vi "GetAvailableDeviceFamilyNames.vi"(8 "Error in":errorcluster) -> (0 "Error out":errorcluster, 2 "Count":i32, 3 "AvailableDeviceFamilies":string[](array[string]))   [LabVIEW 2016]
doc: "Determines a list of all available device families (device drivers).\n\nAvailableDevices: Array of available device family names\nCount: Number of available device families"
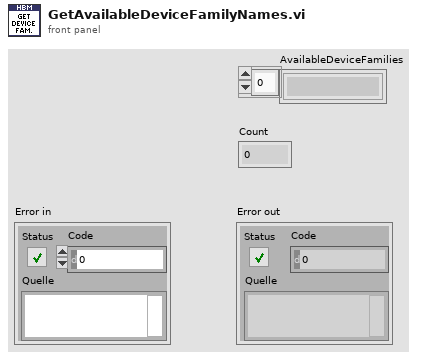
[diagram p1: front panel]
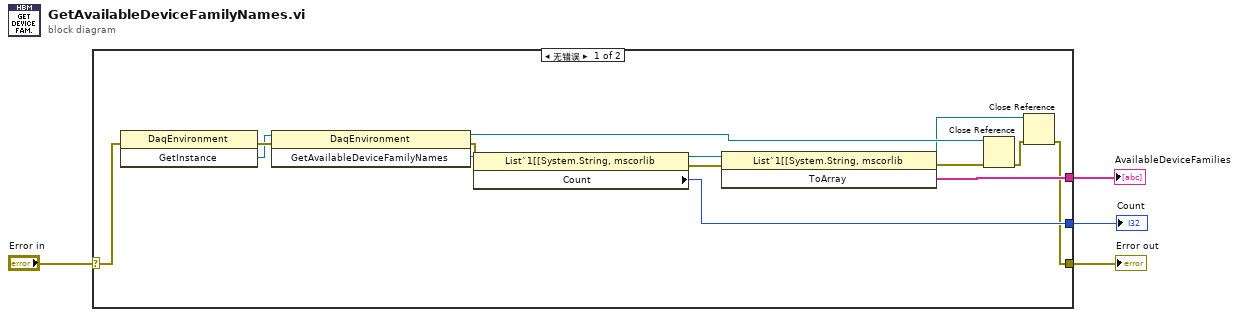
[diagram p0: block diagram]
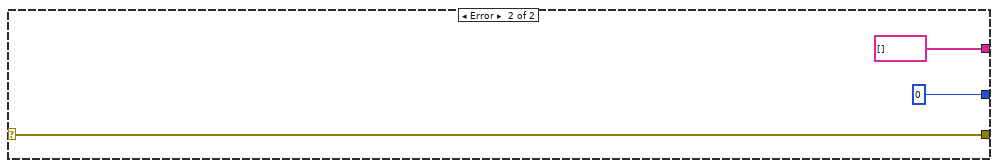
[diagram p2: hidden frame]
diagram:
  n1 = case shown="无错误" "Error in" {
    selector: "Error in" -> [w12 w21]
    tunnel: [w6 w21] -> w3
    tunnel: [w14 string[] [] ("ToArray")] -> w2
    tunnel: [w13 0 ("Count")] -> w1
    frame No Error {
      n2 = invoke on="Methodenknoten" class="DaqEnvironment" method="GetInstance"(error in=w12) -> (error out=w11:errorcluster, "GetInstance"=w10:refnum<k24>)  [unwired: 2 in, 1 out]
      n3 = invoke on="Methodenknoten" class="DaqEnvironment" method="GetAvailableDeviceFamilyNames"(reference=w10, error in=w11) -> (reference out=w8:refnum<k24>, error out=w17:errorcluster, "GetAvailableDeviceFamilyNames"=w18:refnum<k24>)  [unwired: 1 in]
      n4 = property class="List`1[[System.String, mscorlib"(reference=w18, error in=w17) -> (reference out=w16:refnum<k24>, error out=w15:errorcluster, "Count"=w13:i32)
      n5 = invoke class="List`1[[System.String, mscorlib" method="ToArray"(reference=w16, error in=w15) -> (reference out=w5:refnum<k24>, error out=w9:errorcluster, "ToArray"=w14:string[])  [unwired: 1 in]
      n6 = Close Reference(reference=w8, error in (no error)=w9) -> (error out=w7:errorcluster)
      n7 = Close Reference(reference=w5, error in (no error)=w7) -> (error out=w6:errorcluster)
    }
    frame Error {
    }
  }
  "Error out" <- w3
  "AvailableDeviceFamilies" <- w2
  "Count" <- w1
